vi "Start Asynchronous Calls to Array of Transient Captures.vi"(7 "Soft Trigger":bool, 8 "error in":errorcluster, 9 "Pre-Trigger Samples":i32, 10 "Post-Trigger Samples":i32, 11 "List of INI Files":path[](array[path])) -> (0 "error out":errorcluster, 3 "References to Instances":refnum<vi>[](array[refnum]))   [LabVIEW 2017]
doc: "Starts a copy of the transient capture, for each unit under test that is defined by the list of INI files."
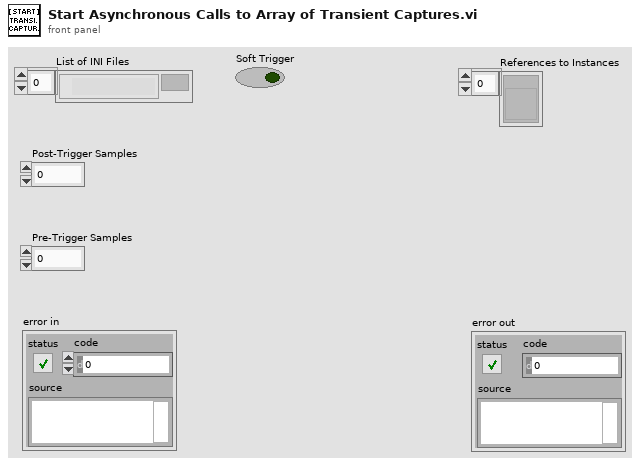
[diagram p1: front panel]
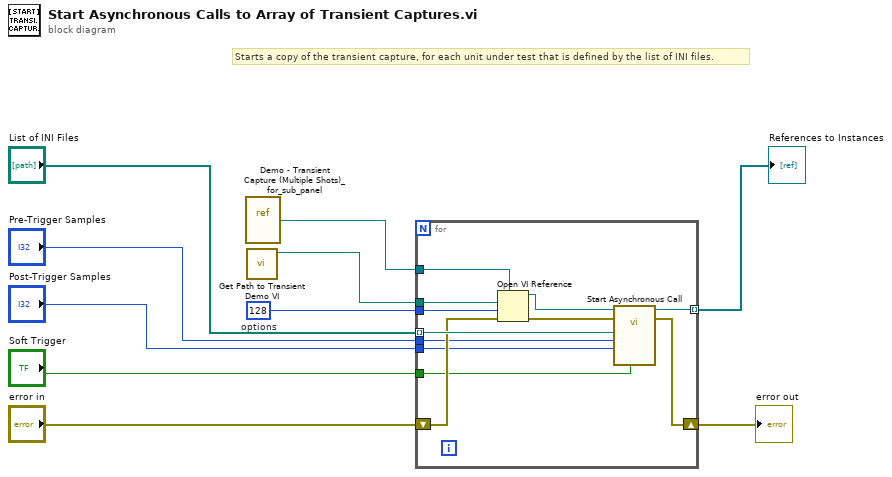
[diagram p0: block diagram]
diagram:
  w8 = 128  # options
  # "Starts a copy of the transient capture, for each unit under test that is defined by the list of INI files."
  n1 = vi-ref "Demo - Transient Capture (Multiple Shots)_for_sub_panel.vi"() -> (w6:refnum<vi>)
  n2 = call "Get Path to Transient Demo VI.vi"() -> ("Path to Transient Capture Subpanel"=w5:path)  [unwired: 11 in]
  n3 = for {
    tunnel: w5 -> [w22]
    tunnel: w6 -> [w21]
    tunnel: "List of INI Files" -> [w18] mode=indexing
    tunnel: [w17] -> w1 mode=indexing
    shift-right: [w16] -> w10
    shift-left: "error in" -> [w14]
    tunnel: w8 -> [w15]
    tunnel: "Soft Trigger" -> [w13]
    tunnel: "Post-Trigger Samples" -> [w12]
    tunnel: "Pre-Trigger Samples" -> [w11]
    n4 = Open VI Reference(type specifier VI Refnum (for type only)=w21, vi path=w22, options=w15, error in (no error)=w14) -> (vi reference=w20:refnum<vi>, error out=w19:errorcluster)  [unwired: 2 in]
    n5 = call-by-ref "Start Asynchronous Call"(reference=w20, error in=w19, "Soft Trigger"=w13, "Post-Trigger Samples"=w12, "Pre-Trigger Samples"=w11, "configuration file path"=w18) -> (reference out=w17:refnum<vi>, error out=w16:errorcluster)  [unwired: 8 in]
  }
  "error out" <- w10
  "References to Instances" <- w1
